vi "Handle mouse enter.vi"(8 "error in (no error)":errorcluster, 11 "Bool D Element in":refnum<class "Bool D Element.lvclass">) -> (0 "error out":errorcluster, 2 "Active cursor":u16, 3 "Bool D Element out":refnum<class "Bool D Element.lvclass">)   [LabVIEW 2020, in "D Datagrid Library.lvlib" / "Bool D Element.lvclass"]
doc: "Sets the mouseover cursor for this element. Override this VI for each child that needs a custom (non-automatic) cursor."
uses:
  Bool D Element.lvclass
  Bool D Element.lvclass/Bool D Element.ctl
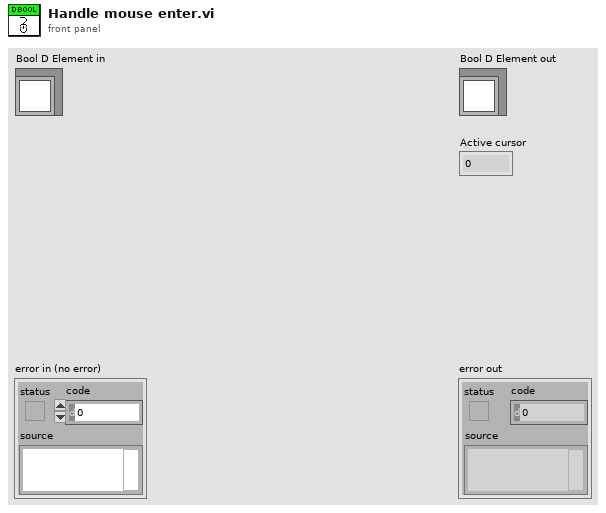
[diagram p1: front panel]
types:
  T1 = typedef "LVFontTypeDef.ctl" = cluster{"Font Name":string, "Size":u16, "Bold":bool, "Italic":bool, "Underline":bool, "Strikeout":bool, "Color":u32}
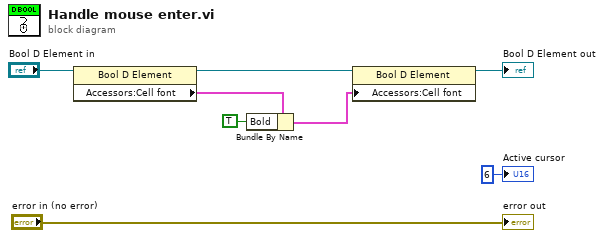
[diagram p0: block diagram]
diagram:
  n1 = property class="Bool D Element"(reference="Bool D Element in") -> (reference out=w5:refnum<class "Bool D Element.lvclass">, "Accessors:Cell font"=w3:T1)  [unwired: 1 in, 1 out]
  n2 = Bundle By Name(cluster=w3, "Bold"=TRUE) -> (w2:T1)
  n3 = property class="Bool D Element"(reference=w5, "Accessors:Cell font"=w2) -> (reference out=→"Bool D Element out":refnum<class "Bool D Element.lvclass">)  [unwired: 1 in, 1 out]
  "error out" <- "error in (no error)"
  "Active cursor" <- u16 6 ("Active cursor")
